vi "Power Case Statement.vi"() -> ()   [LabVIEW 2018]
panel:
  out "String":string
  in  "Slide":i32(slide) scale=-5.0..15.0
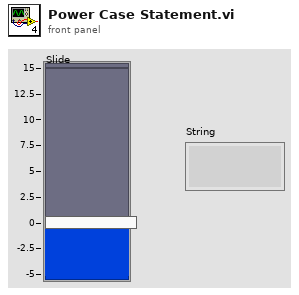
[diagram p1: front panel]
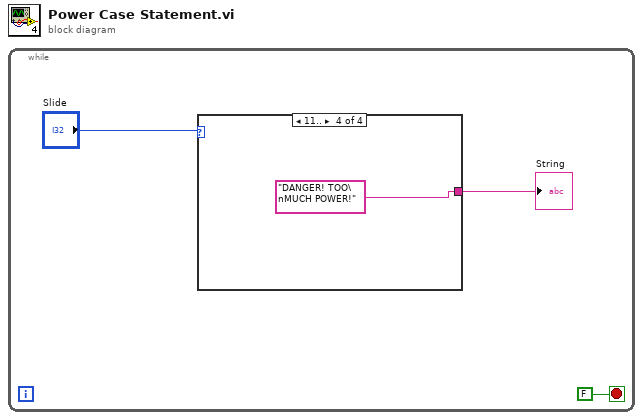
[diagram p0: block diagram]
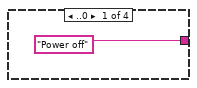
[diagram p2: hidden frame]
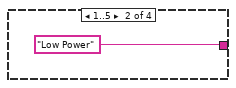
[diagram p3: hidden frame]
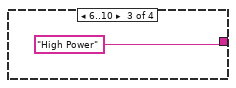
[diagram p4: hidden frame]
diagram:
  n1 = while {
    stop <- FALSE stop-if-true
    n2 = case shown="11.." "Slide" {
      tunnel: ["Power off" "Low Power" "High Power" "DANGER! TOO\nMUCH POWER!"] -> w2
      frame ..0 {
      }
      frame 1..5 {
      }
      frame 6..10 {
      }
      frame 11.. {
      }
    }
    "String" <- w2
  }
